vi "M-686 Wait for Action.vi"(0 "M686 Note":refnum<notifier>, 11 "Error In":errorcluster) -> (4 "Note Out":refnum<notifier>, 15 "Error Out":errorcluster)   [LabVIEW 2020]
uses:
  Stages Controls/Stage Notifier Element.ctl
  Stages Controls/Stage Actions.ctl
  Stages Controls/Stage Status.ctl
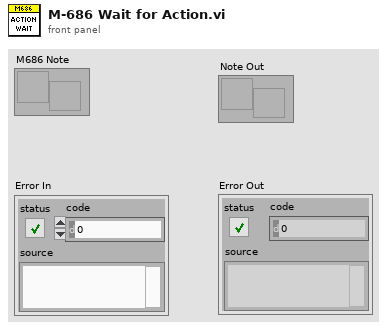
[diagram p1: front panel]
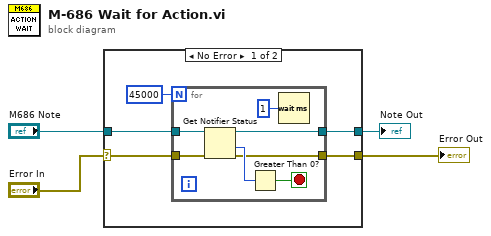
[diagram p0: block diagram]
diagram:
  n1 = case shown="No Error" "Error In" {
    selector: "Error In" -> [w7 w17]
    tunnel: "M686 Note" -> [w9 w18]
    tunnel: [w6 w18] -> w2
    tunnel: [w5 w17] -> w1
    frame No Error {
      n2 = for {
        N: 45000 -> [_]
        tunnel: w9 -> [w16]
        tunnel: w7 -> [w13]
        tunnel: [w12] -> w6
        tunnel: [w11] -> w5
        stop <- w14 stop-if-true
        n3 = Get Notifier Status(notifier=w16, error in (no error)=w13) -> (notifier out=w12:refnum<notifier>, # waiting=w15:i32, error out=w11:errorcluster)  [unwired: 2 out]
        n4 = Greater Than 0?(x=w15) -> (x > 0?=w14:bool)
        n5 = Wait (ms)(milliseconds to wait=u32 1) -> ()  [unwired: 1 out]
      }
    }
    frame Error {
    }
  }
  "Note Out" <- w2
  "Error Out" <- w1
